vi "Start Display Routine.vi"(8 "error in":errorcluster, 9 "starting address":u16, 10 "register to write":u16, 11 "Modbus master in":refnum<class "Modbus Master.lvclass">) -> (0 "error out":errorcluster, 2 "register values":u16[](array[numeric]), 3 "Modbus master out":refnum<class "Modbus Master.lvclass">)   [LabVIEW 2023]
uses:
  <vilib>/NI/Modbus Library/API/Master/Modbus Master.lvclass
  RS485/RS485.lvlib
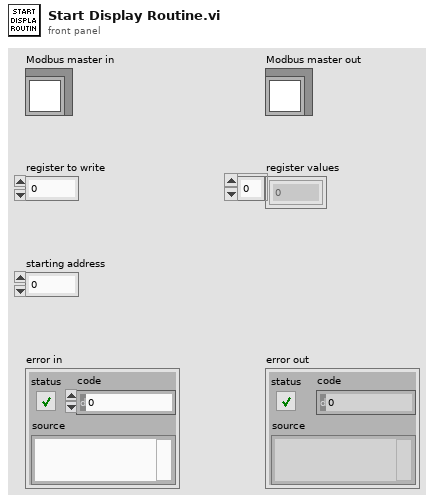
[diagram p1: front panel]
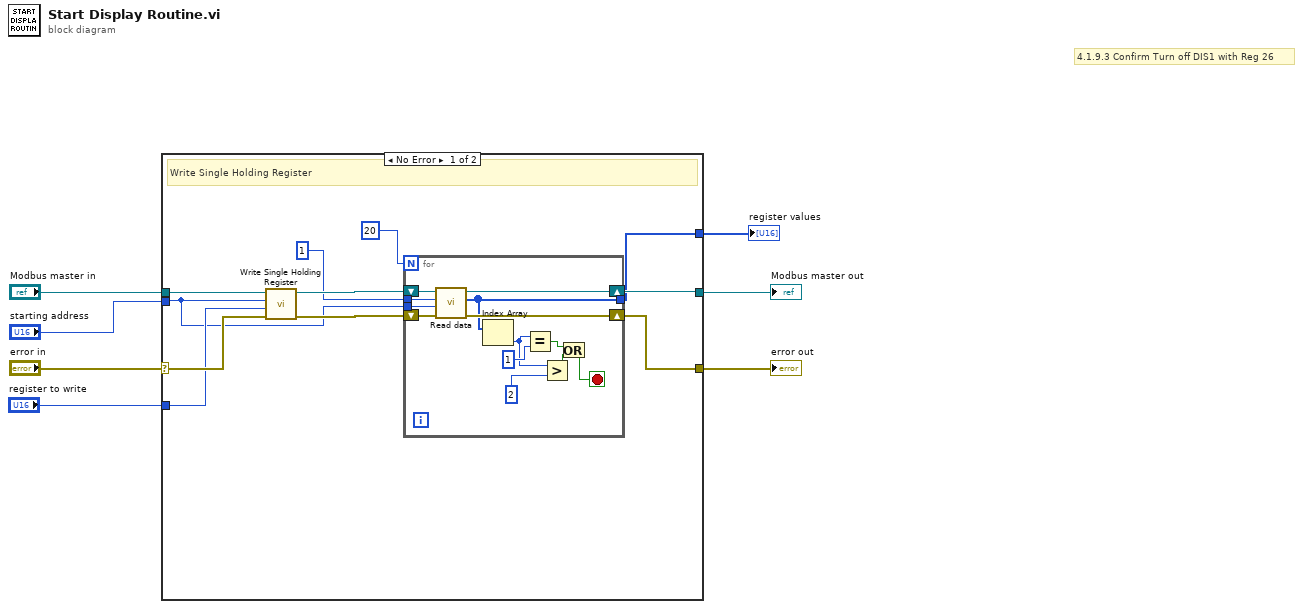
[diagram p0: block diagram]
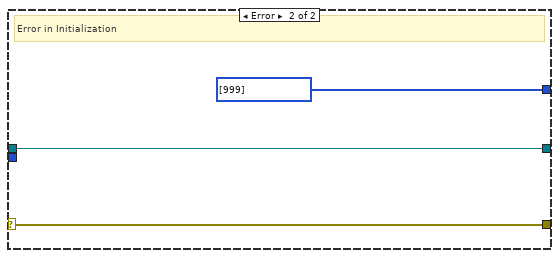
[diagram p2: hidden frame]
diagram:
  # "4.1.9.3 Confirm Turn off DIS1 with Reg 26"
  n1 = case shown="No Error" "error in" {
    selector: "error in" -> [w17 w33]
    tunnel: "Modbus master in" -> [w18 w34]
    tunnel: [w14 w34] -> w4
    tunnel: [w12 w33] -> w3
    tunnel: "starting address" -> [w10 _]
    tunnel: "register to write" -> [w16 _]
    tunnel: [w9 u16[] [999] ("register values")] -> w1
    frame No Error {
      # "Write Single Holding Register"
      n2 = call-dynamic "Write Single Holding Register.vi"("error in"=w17, "register to write"=w16, "address"=w10, "Modbus master in"=w18) -> ("error out"=w13:errorcluster, "Modbus master out"=w15:refnum<class "Modbus Master.lvclass">)  [unwired: 6 in]
      n3 = for {
        N: 20 -> [_]
        tunnel: u16 1 ("number of inputs") -> [w27]
        tunnel: w10 -> [w26]
        tunnel: [w25] -> w9
        shift-right: [w30] -> w14
        shift-left: w15 -> [w31]
        shift-right: [w28] -> w12
        shift-left: w13 -> [w29]
        stop <- w22 stop-if-true
        n4 = call "Read data.vi"("error in"=w29, "starting address"=w26, "number of inputs"=w27, "Modbus master in"=w31) -> ("error out"=w28:errorcluster, "register values"=w25:u16[], "Modbus master out"=w30:refnum<class "Modbus Master.lvclass">)  [unwired: 5 in]
        n5 = Index Array(array=w25) -> (element=w21:u16)  [unwired: 1 in]
        n6 = Equal?(x=w21, y=u16 1) -> (x = y?=w23:bool)
        n7 = Greater?(x=w21, y=u16 2) -> (0:w19:bool)
        n8 = Or(x=w23, y=w19) -> (x .or. y?=w22:bool)
      }
    }
    frame Error {
      # "Error in Initialization"
    }
  }
  "Modbus master out" <- w4
  "error out" <- w3
  "register values" <- w1
